vi "Set Task.vi"(8 "error in (no error)":errorcluster caption="entrée d'erreur (pas d'erreur)", 10 "Task":refnum<k21>, 11 "Class DIO NI en entrée":refnum<class "Class Ana NI.lvclass">) -> (0 "error out":errorcluster caption="sortie d'erreur", 3 "Class DIO NI en sortie":refnum<class "Class Ana NI.lvclass">)   [LabVIEW 2020, in "Library Instrument & Equipement.lvlib" / "Library Ana.lvlib" / "Class Ana NI.lvclass"]
uses:
  Class Ana NI.lvclass
  Class Ana NI.lvclass/Class Ana NI.ctl
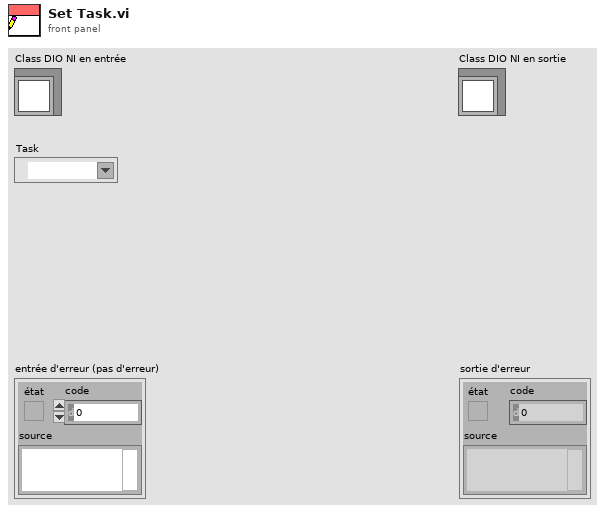
[diagram p1: front panel]
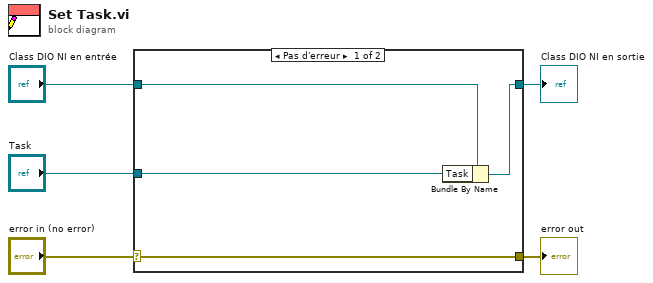
[diagram p0: block diagram]
diagram:
  n1 = case shown="Pas d'erreur" "error in (no error)" {
    selector: "error in (no error)" -> [w9 w10]
    tunnel: [w9 w10] -> w4
    tunnel: [w7 w11] -> w2
    tunnel: "Class DIO NI en entrée" -> [w8 w11]
    tunnel: "Task" -> [w6 _]
    frame No Error {
      n2 = Bundle By Name(cluster=w8, "Task"=w6) -> (w7:refnum<class "Class Ana NI.lvclass">)
    }
    frame Error {
    }
  }
  "error out" <- w4
  "Class DIO NI en sortie" <- w2
